vi "Read Init.vi"(8 "error in (no error)":errorcluster, 11 "Valve Controller in":refnum<class "Valve Controller.lvclass">) -> (0 "error out":errorcluster, 2 "Init":bool, 3 "Valve Controller out":refnum<class "Valve Controller.lvclass">)   [LabVIEW 2011, in "Valve Controller.lvclass"]
uses:
  Valve Controller.lvclass
  Valve Controller.lvclass/Valve Controller.ctl
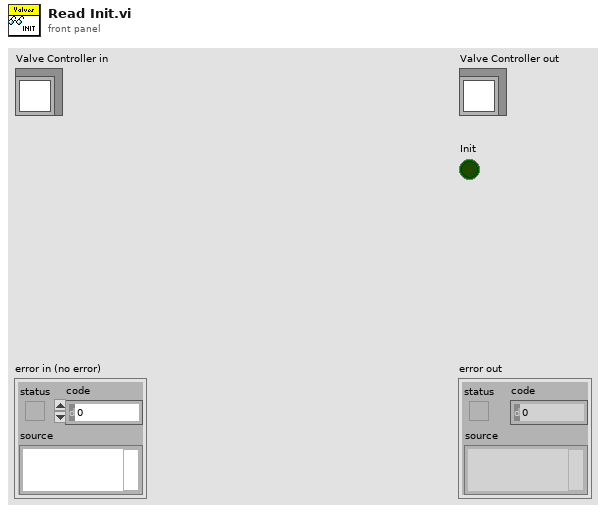
[diagram p1: front panel]
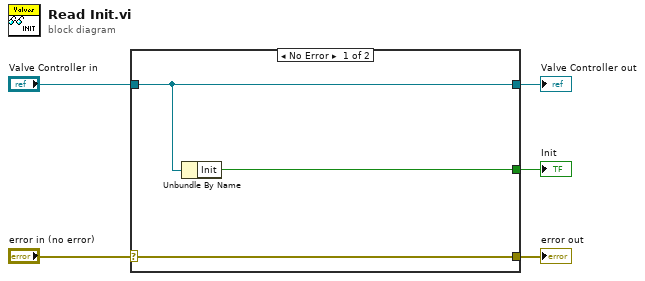
[diagram p0: block diagram]
diagram:
  n1 = case shown="No Error" "error in (no error)" {
    selector: "error in (no error)" -> [w8 w9]
    tunnel: [w8 w9] -> w4
    tunnel: [w7 w10] -> w2
    tunnel: "Valve Controller in" -> [w7 w10]
    tunnel: [w6 _] -> w1
    frame No Error {
      n2 = Unbundle By Name(w7) -> ("Init"=w6:bool)
    }
    frame Error {
    }
  }
  "error out" <- w4
  "Valve Controller out" <- w2
  "Init" <- w1
